vi "Delay.vi"(8 "error in (no error)":errorcluster, 10 "Delay Time (10)":u32=10, 11 "VISA resource name":refnum<visa-resource-name>) -> (0 "error out":errorcluster, 3 "VISA resource name out":refnum<visa-resource-name>)   [LabVIEW 2015, in "SDG X Series.lvlib"]
doc: "Creates a time delay in milliseconds."
uses:
  <instrlib>/SDG X Series/SDG X Series.lvlib
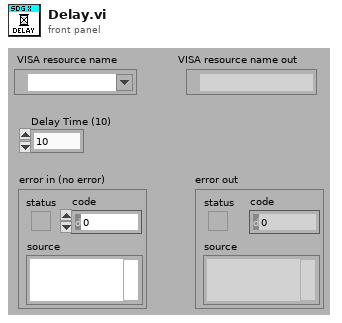
[diagram p1: front panel]
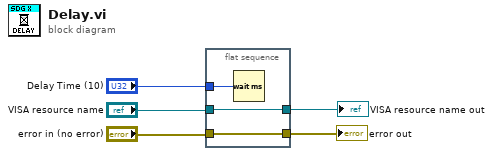
[diagram p0: block diagram]
diagram:
  n1 = flat-sequence {
    tunnel: [w8] -> w2
    tunnel: "VISA resource name" -> [w8]
    tunnel: "error in (no error)" -> [w7]
    tunnel: [w7] -> w3
    tunnel: "Delay Time (10)" -> [w6]
    frame #0 {
      n2 = Wait (ms)(milliseconds to wait=w6) -> ()  [unwired: 1 out]
    }
  }
  "VISA resource name out" <- w2
  "error out" <- w3
